vi "Remove Non-Numeric Columns.vi"(1 "Separator (Tab)":string="\t", 2 "String In":string="       \t8/25/2005\t6:01 PM\t   0.10\t   0.20\t   0.30\t   0.40\r\n   V   \t8/25/2005\t6:02 PM\t   1.10\t   1.20\t   1.30\t   1.40\r\n       \t8/25/2005\t6:03 PM\t   2.10\t   2.20\t   2.30\t   2.40\r\n       \t8/25/2005\t6:04 PM\t   3.10\t   3.20\t   3.30\t   3.40\r\n   V   \t8/25/2005\t6:05 PM\t   4.10\t   4.20\t   4.30\t   4.40\r\n", 4 "Remove Columns":i32[](array[numeric])=[1, 2, 3]) -> (6 "Removed Columns":string[][](array[string]), 7 "String Out":string)   [LabVIEW 2013]
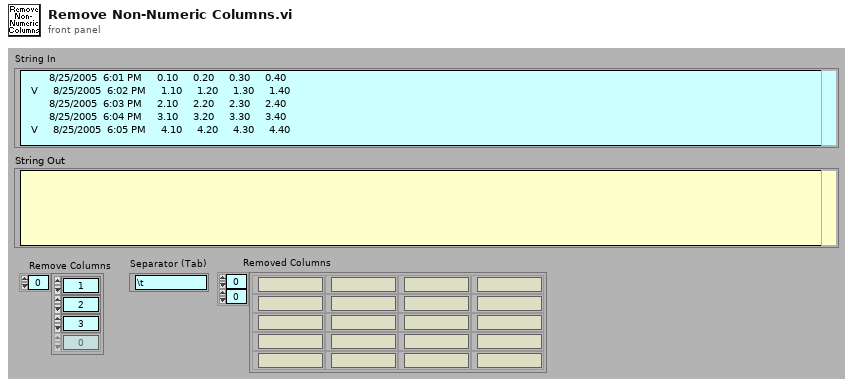
[diagram p1: front panel]
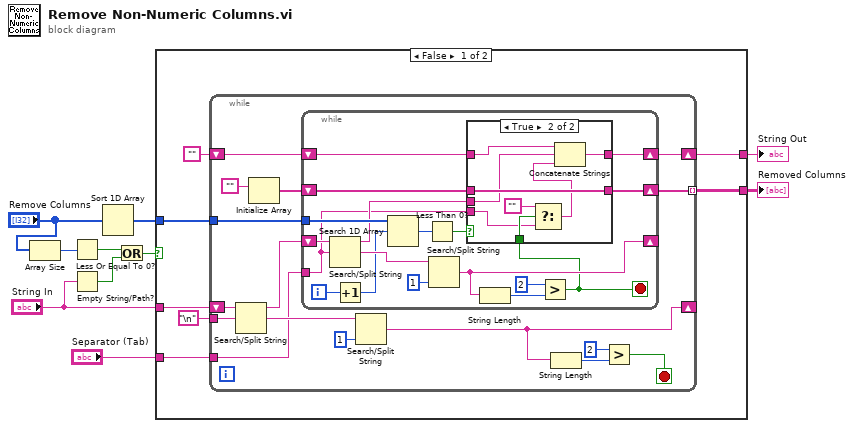
[diagram p0: block diagram]
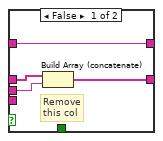
[diagram p2: hidden frame]
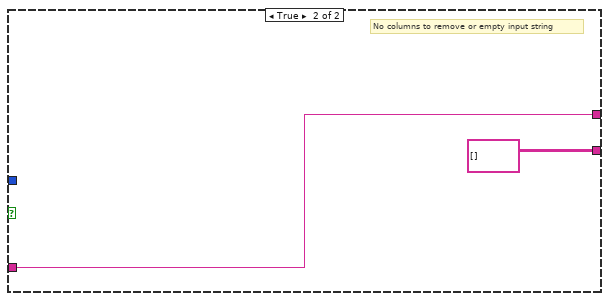
[diagram p3: hidden frame]
diagram:
  n1 = Array Size(array="Remove Columns") -> (size(s)=w10:i32)
  n2 = Less Or Equal To 0?(x=w10) -> (x <= 0?=w9:bool)
  n3 = Empty String/Path?(string/path="String In") -> (empty?=w8:bool)
  n4 = Sort 1D Array(array="Remove Columns") -> (sorted array=w2:i32[])
  n5 = Or(x=w9, y=w8) -> (x .or. y?=w5:bool)
  n6 = case shown="False" w5 {
    tunnel: "String In" -> [w17 w65]
    tunnel: [w14 w65] -> w6
    tunnel: [w15 string[][] [] ("Removed Columns")] -> w4
    tunnel: w2 -> [w13 _]
    tunnel: "Separator (Tab)" -> [w16 _]
    frame False {
      n7 = while {
        shift-right: [w18] -> _
        shift-left: w17 -> [w33]
        tunnel: "\n" -> [w32]
        tunnel: w13 -> [w26]
        tunnel: w16 -> [w27]
        tunnel: [w23] -> w15 mode=indexing
        shift-right: [w21] -> w14
        shift-left: "" -> [w22]
        stop <- w29 stop-if-true
        n8 = Search/Split String(string=w33, search string/char (-)=w32) -> (substring before match=w28:string, match + rest of string=w31:string)  [unwired: 1 in, 1 out]
        n9 = Initialize Array("") -> (w25:string[])  [unwired: 1 in]
        n10 = while {
          shift-right: [w39] -> _
          shift-left: w28 -> [w51]
          tunnel: w27 -> [w36]
          tunnel: w26 -> [w47]
          shift-right: [w41] -> w23
          shift-left: w25 -> [w42]
          shift-right: [w35] -> w21
          shift-left: w22 -> [w40]
          i -> [w50]
          stop <- w34 stop-if-true
          n11 = Search/Split String(string=w51, search string/char (-)=w36) -> (substring before match=w43:string, match + rest of string=w48:string)  [unwired: 1 in, 1 out]
          n12 = Increment(x=w50) -> (x+1=w46:i32)
          n13 = Search 1D Array(1D array=w47, element=w46) -> (index of element=w45:i32)  [unwired: 1 in]
          n14 = Less Than 0?(x=w45) -> (x < 0?=w44:bool)
          n15 = Search/Split String(string=w48, offset (0)=1) -> (match + rest of string=w39:string)  [unwired: 1 in, 2 out]
          n16 = String Length(string=w39) -> (length=w38:i32)
          n17 = Greater?(x=2 ("y"), y=w38) -> (0:w34:bool)
          n18 = case shown="True" w44 {
            tunnel: w43 -> [w53 w58]
            tunnel: w42 -> [w55 w63]
            tunnel: [w54 w63] -> w41
            tunnel: w40 -> [w52 w62]
            tunnel: [w52 w61] -> w35
            tunnel: w36 -> [_ w57]
            tunnel: w34 -> [_ w59]
            frame False {
              # "Remove\nthis col"
              n19 = Build Array (concatenate)(w55, w53) -> (w54:string[])
            }
            frame True {
              n20 = Select(t="", s=w59, f=w57) -> (s? t:f=w56:string)
              n21 = Concatenate Strings(w62, w58, w56) -> (w61:string)
            }
          }
        }
        n22 = Search/Split String(string=w31, offset (0)=1) -> (match + rest of string=w18:string)  [unwired: 1 in, 2 out]
        n23 = String Length(string=w18) -> (length=w20:i32)
        n24 = Greater?(x=2 ("y"), y=w20) -> (0:w29:bool)
      }
    }
    frame True {
      # "No columns to remove or empty input string"
    }
  }
  "String Out" <- w6
  "Removed Columns" <- w4
